vi "Part 2.vi"(11 "Input":string) -> (3 "Output":i64)   [LabVIEW 2021]
uses:
  <userlib>/_OpenG.lib/string/string.llb/Convert EOLs (String)__ogtk.vi
panel:
  in  "Tab Control":enum32{"Graph", "Intensity"}(tab)
  out "Lines":cluster{cluster{i32, i32}[]}[](graph)
  out "Grid":i64[][](graph)
  out "min y":i32
  out "max y":i32
  out "min x":i32
  out "max x":i32
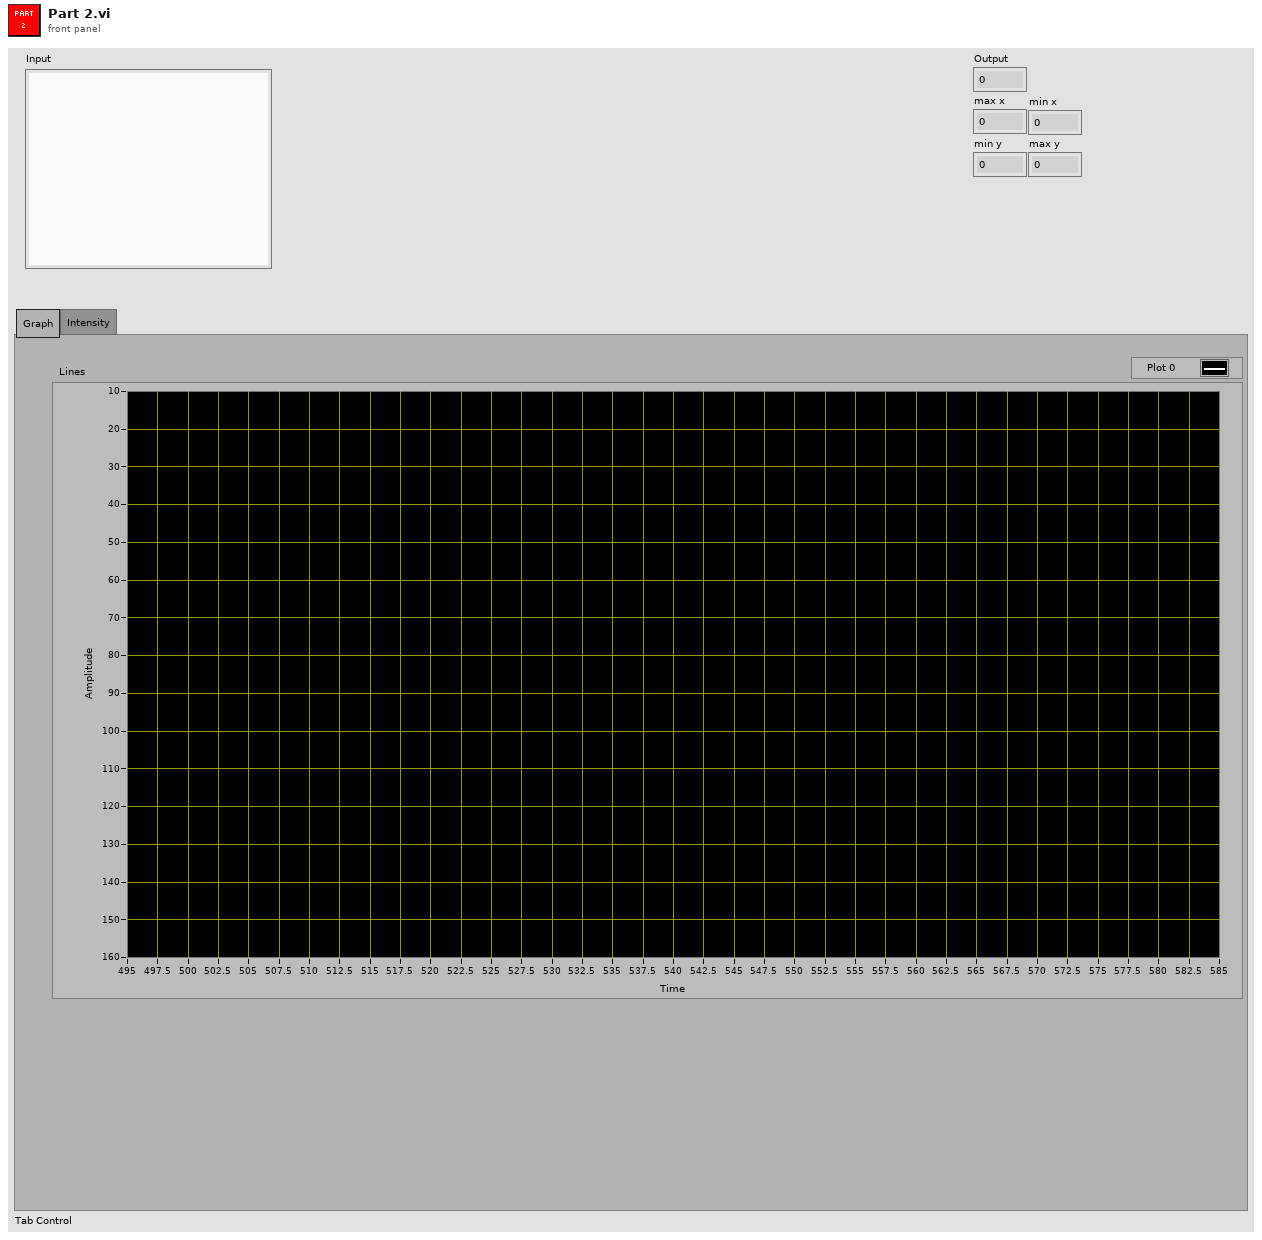
[diagram p1: front panel]
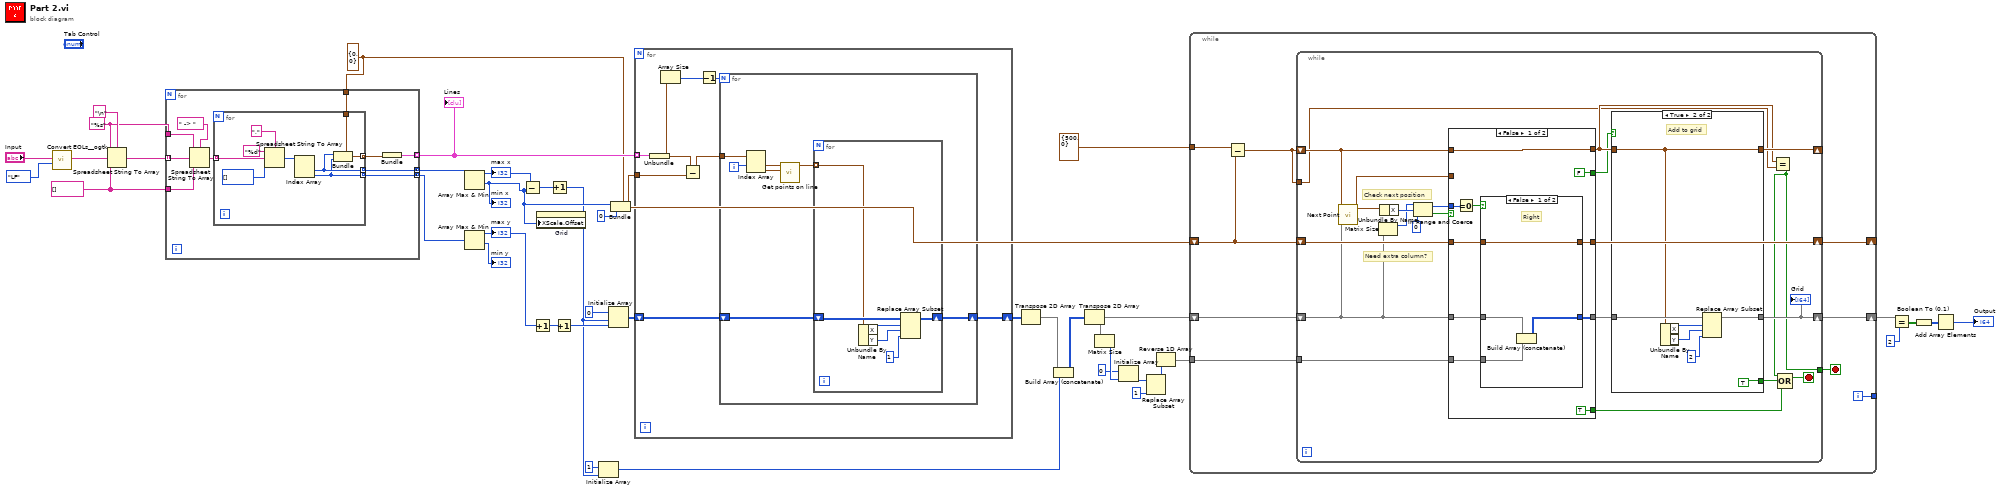
[diagram p0: block diagram]
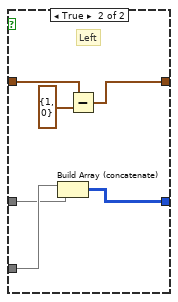
[diagram p2: hidden frame]
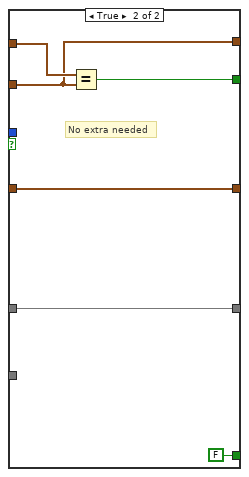
[diagram p3: hidden frame]
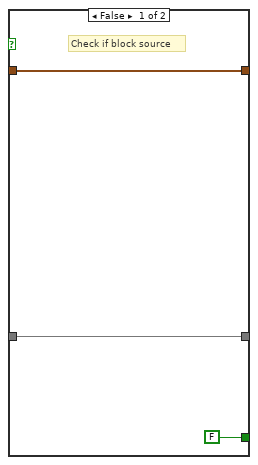
[diagram p4: hidden frame]
diagram:
  w22 = cluster{"X":i32, "Y":i32} {"X"=0, "Y"=0} ("cluster")
  w35 = string[] []
  w36 = "%s"
  n1 = call-poly <userlib>:"Convert EOLs__ogtk.vi"("Convert to:"=enum16{"CR", "LF", "CRLF"}."LF", "String in"="Input") -> ("String out"=w39:string)  [unwired: 9 in]
  n2 = Spreadsheet String To Array(delimiter (Tab)="\n", format string=w36, spreadsheet string=w39, array type (2D Dbl)=w35) -> (array=w37:string[])
  n3 = for {
    tunnel: w37 -> [w49] mode=indexing
    tunnel: w36 -> [w51]
    tunnel: w35 -> [w50]
    tunnel: [w46] -> w32 mode=concatenating
    tunnel: [w45] -> w33 mode=concatenating
    tunnel: [w43] -> w27 mode=indexing
    tunnel: w22 -> [w42]
    n4 = Spreadsheet String To Array(delimiter (Tab)=" -> ", format string=w51, spreadsheet string=w49, array type (2D Dbl)=w50) -> (array=w47:string[])
    n5 = for {
      tunnel: w47 -> [w60] mode=indexing
      tunnel: [w55] -> w46 mode=indexing
      tunnel: [w54] -> w45 mode=indexing
      tunnel: [w53] -> w44 mode=indexing
      tunnel: w42 -> [w52]
      n6 = Spreadsheet String To Array(delimiter (Tab)=",", format string="%d", spreadsheet string=w60, array type (2D Dbl)=i32[] []) -> (array=w56:i32[])
      n7 = Index Array(array=w56) -> (element #1=w55:i32, element #2=w54:i32)  [unwired: 2 in]
      n8 = Bundle(cluster=w52, "X"=w55, "Y"=w54) -> (w53:cluster{"X":i32, "Y":i32})
    }
    n9 = Bundle(w44) -> (w43:cluster{cluster{"X":i32, "Y":i32}[]})  [unwired: 1 in]
  }
  "Lines" <- w27
  n10 = Array Max & Min(array=w32) -> (max value=w31:i32, min value=w25:i32)  [unwired: 2 out]
  "max x" <- w31
  "min x" <- w25
  n11 = Array Max & Min(array=w33) -> (max value=w26:i32, min value=→"min y":i32)  [unwired: 2 out]
  "max y" <- w26
  n12 = Subtract(x=w31, y=w25) -> (x-y=w30:i32)
  n13 = Increment(x=w26) -> (x+1=w13:i32)
  n14 = property on="Grid" class="IntGraph (strict)"("XScale.Offset"=w25) -> ()  [unwired: 2 in, 2 out]
  n15 = Increment(x=w30) -> (x+1=w14:i32)
  n16 = Increment(x=w13) -> (x+1=w24:i32)
  n17 = Initialize Array(i64 1 ("element"), w14) -> (w18:i64[])
  n18 = Initialize Array(i64 0 ("element"), w14, w24) -> (w28:i64[][])
  n19 = Bundle(cluster=w22, "X"=w25, "Y"=0 ("min x")) -> (w20:cluster{"X":i32, "Y":i32})
  n20 = for {
    shift-right: [w64] -> w17
    shift-left: w28 -> [w65]
    tunnel: w27 -> [w68] mode=indexing
    tunnel: w20 -> [w61]
    n21 = Unbundle(w68) -> (w63:cluster{"X":i32, "Y":i32}[])
    n22 = Array Size(array=w63) -> (size(s)=w67:i32)
    n23 = Subtract(x=w63, y=w61) -> (x-y=w62:cluster{"X":i32, "Y":i32}[])
    n24 = Decrement(x=w67) -> (x-1=w66:i32)
    n25 = for {
      N: w66 -> [_]
      tunnel: w62 -> [w75]
      shift-right: [w69] -> w64
      shift-left: w65 -> [w70]
      i -> [w74]
      n26 = Index Array(array=w75, index #1=w74) -> (element #1=w73:cluster{"X":i32, "Y":i32}, element #2=w72:cluster{"X":i32, "Y":i32})  [unwired: 1 in]
      n27 = call "Get points on line.vi"("Stop"=w72, "Start"=w73) -> ("Line"=w71:cluster{"X":i32, "Y":i32}[])  [unwired: 9 in]
      n28 = for {
        tunnel: w71 -> [w79] mode=indexing
        shift-right: [w80] -> w69
        shift-left: w70 -> [w81]
        n29 = Unbundle By Name(w79) -> ("X"=w78:i32, "Y"=w77:i32)
        n30 = Replace Array Subset(array=w81, new element=i64 1 ("new element/subarray"), index (row)=w78, index (col)=w77) -> (w80:i64[][])
      }
    }
  }
  n31 = Transpose 2D Array(2D array=w17) -> (transposed array=w15:i64[][])
  n32 = Build Array (concatenate)(w15, w18) -> (w16:i64[][])
  n33 = Transpose 2D Array(2D array=w16) -> (transposed array=w12:i64[][])
  n34 = Matrix Size(0:w12) -> (2:w11:i32)  [unwired: 1 out]
  n35 = Initialize Array(0 ("lower limit"), w11) -> (w9:i32[])
  n36 = Replace Array Subset(array=w9, new element=1 ("new element/subarray")) -> (w7:i32[])  [unwired: 1 in]
  n37 = Reverse 1D Array(array=w7) -> (reversed array=w6:i32[])
  n38 = while {
    shift-right: [w89] -> w5
    shift-left: w12 -> [w90]
    tunnel: [w88] -> _
    tunnel: cluster{"X":i32, "Y":i32} {"X"=500, "Y"=0} ("Rest") -> [w86]
    shift-right: [w83] -> _
    shift-left: w20 -> [w84]
    tunnel: w6 -> [w82]
    i -> [w88]
    stop <- w87 stop-if-true
    n39 = Subtract(x=w86, y=w84) -> (x-y=w85:cluster{"X":i32, "Y":i32})
    n40 = while {
      shift-right: [w110] -> w89
      shift-left: w90 -> [w101]
      shift-right: [w109] -> _
      shift-left: w85 -> [w96]
      tunnel: [w92] -> w87
      tunnel: w85 -> [w93]
      shift-right: [w102] -> w83
      shift-left: w84 -> [w103]
      tunnel: w82 -> [w98]
      stop <- w111 stop-if-true
      # "Need extra column?"
      # "Check next position"
      n41 = call "Next Point.vi"("Grid In"=w101, "Point"=w96) -> ("Point out"=w97:cluster{"X":i32, "Y":i32})  [unwired: 9 in]
      n42 = Matrix Size(0:w101) -> (1:w106:i32)  [unwired: 1 out]
      n43 = Unbundle By Name(w97) -> ("X"=w107:i32)
      n44 = In Range and Coerce(upper limit=w106, x=w107, lower limit=0) -> (coerced(x)=w99:i32, In Range?=w104:bool)
      n45 = case shown="False" w104 {
        tunnel: w103 -> [w116 w137]
        tunnel: [w117 w137] -> w102
        tunnel: w101 -> [w119 w136]
        tunnel: [w118 w136] -> w100
        tunnel: w99 -> [w121 _]
        tunnel: w98 -> [w115 _]
        tunnel: w97 -> [_ w133]
        tunnel: w96 -> [w113 w134]
        tunnel: [FALSE w135] -> w94
        tunnel: [w113 w133] -> w95
        tunnel: [TRUE FALSE] -> w91
        frame False {
          n46 = Equal To 0?(x=w121) -> (x = 0?=w120:bool)
          n47 = case shown="False" w120 {
            tunnel: w119 -> [w122 w129]
            tunnel: [w123 w130] -> w118
            tunnel: [w125 w128] -> w117
            tunnel: w116 -> [w125 w127]
            tunnel: w115 -> [w124 w131]
            frame False {
              # "Right"
              n48 = Build Array (concatenate)(w122, w124) -> (w123:i64[][])
            }
            frame True {
              # "Left"
              n49 = Build Array (concatenate)(w131, w129) -> (w130:i64[][])
              n50 = Subtract(x=w127, y=cluster{"X":i32, "Y":i32} {"X"=1, "Y"=0}) -> (x-y=w128:cluster{"X":i32, "Y":i32})
            }
          }
        }
        frame True {
          # "No extra needed"
          n51 = Equal?(x=w134, y=w133) -> (x = y?=w135:bool)
        }
      }
      n52 = case shown="True" w94 {
        tunnel: w95 -> [w138 w141]
        tunnel: w100 -> [w139 w143]
        tunnel: [w139 w142] -> w110
        tunnel: [w138 w141] -> w109
        tunnel: [FALSE TRUE] -> w108
        frame False {
          # "Check if block source"
        }
        frame True {
          # "Add to grid"
          n53 = Unbundle By Name(w141) -> ("X"=w146:i32, "Y"=w145:i32)
          n54 = Replace Array Subset(array=w143, new element=i64 2 ("new element/subarray"), index (row)=w146, index (col)=w145) -> (w142:i64[][])
        }
      }
      "Grid" <- w110
      n55 = Equal?(x=w95, y=w93) -> (x = y?=w92:bool)
      n56 = Compound Arithmetic op=OR(w92, w108, w91) -> (w111:bool)
    }
  }
  n57 = Equal?(x=w5, y=i64 2 ("new element/subarray")) -> (x = y?=w3:bool[][])
  n58 = Boolean To (0,1)(Boolean=w3) -> (0, 1=w2:i16[][])
  n59 = Add Array Elements(numeric array=w2) -> (sum=→"Output":i16)
